vi "AddCurrentSweep.vi"(0 "deviceName":string, 1 "quietTimeSamplingInterval":sgl=1.0, 2 "endingCurrent":sgl, 3 "samplingInterval":sgl, 5 "channel":u8, 7 "repeats":u16=1, 8 "alphaFactor":sgl=75.0, 9 "quietTime":sgl, 10 "minVoltage":sgl=-inf, 11 "error in (no error)":errorcluster, 12 "startingCurrent":sgl, 13 "scanRate":sgl, 14 "maxVoltage":sgl=inf) -> (15 "error out":errorcluster)   [LabVIEW 2018]
doc: "EXPORT void AisAddCurrentSweep(const char* deviceName, uint8_t channel, uint16_t repeats, float quietTime, float quietTimeSamplingInterval, float startingCurrent, float endingCurrent, float scanRate, float samplingInterval, float maxVoltage, float minVoltage, float alphaFactor);"
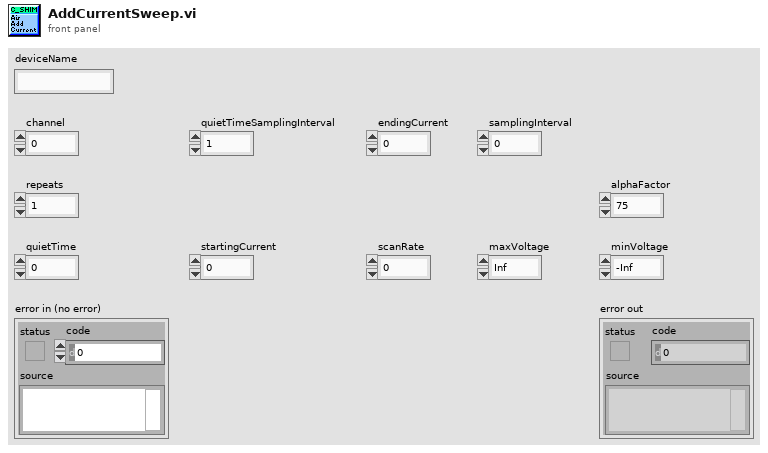
[diagram p1: front panel]
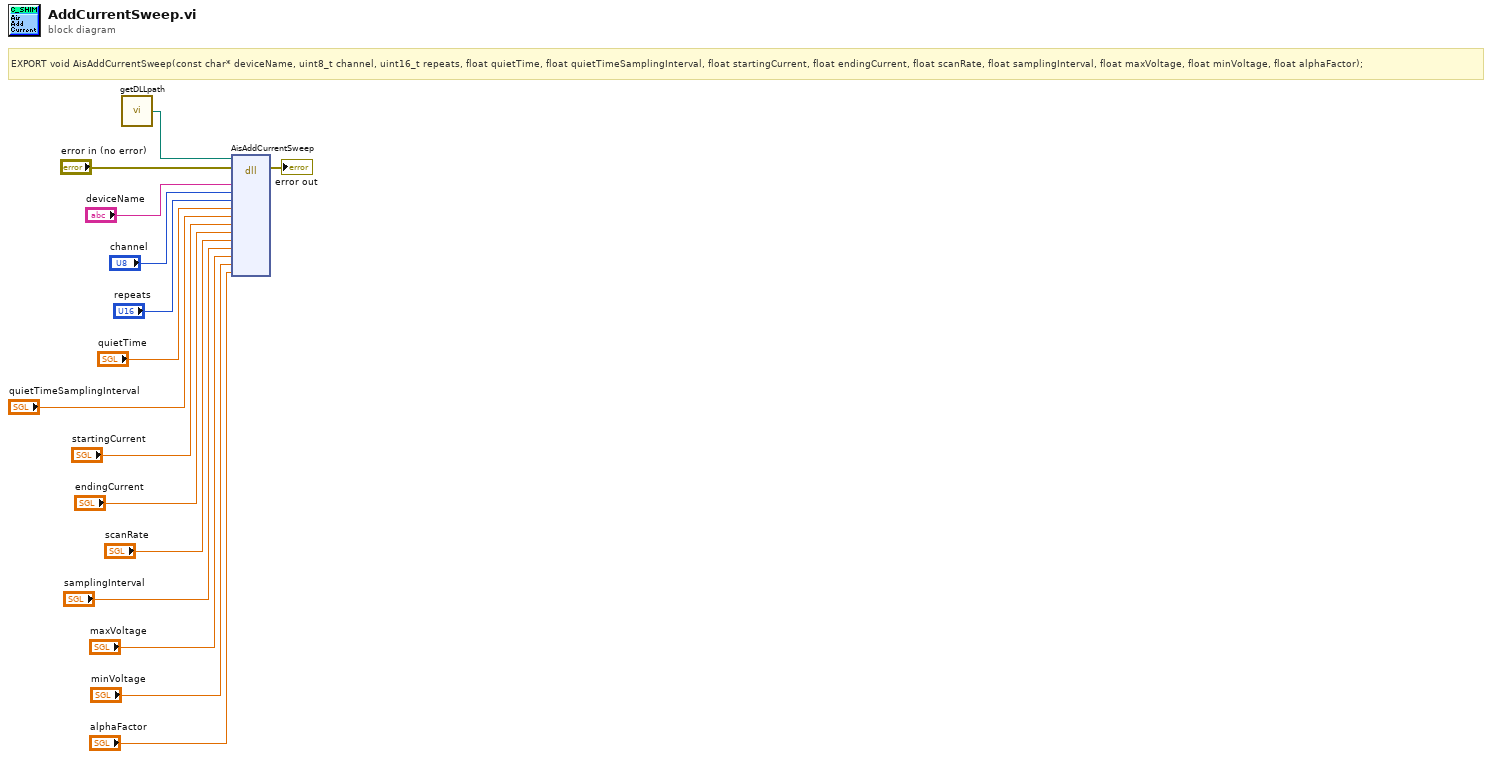
[diagram p0: block diagram]
diagram:
  # "EXPORT void AisAddCurrentSweep(const char* deviceName, uint8_t channel, uint16_t repeats, float quietTime, float quietTimeSamplingInterval, float startingCurrent, float endingCurrent, float scanRate, float samplingInterval, float maxVoltage, float minVoltage, float alphaFactor);"
  n1 = call "getDLLpath.vi"() -> ("DLL_Path"=w1:path)
  n2 = dll-call lib="?" fn="AisAddCurrentSweep"(path in=w1, error in="error in (no error)", "deviceName"="deviceName", "channel"="channel", "repeats"="repeats", "quietTime"="quietTime", "quietTimeSamplingInterval"="quietTimeSamplingInterval", "startingCurrent"="startingCurrent", "endingCurrent"="endingCurrent", "scanRate"="scanRate", "samplingInterval"="samplingInterval", "maxVoltage"="maxVoltage", "minVoltage"="minVoltage", "alphaFactor"="alphaFactor") -> (error out=→"error out":errorcluster)  [unwired: 14 in, 1 out]
